vi "Read resource name.vi"(8 "error in (no error)":errorcluster, 11 "FPGATarget in":refnum<class "FPGATarget.lvclass">) -> (0 "error out":errorcluster, 2 "RIO Device":T1, 3 "FPGATarget out":refnum<class "FPGATarget.lvclass">)   [LabVIEW 2013, in "FPGATarget.lvclass"]
uses:
  FPGATarget.lvclass
  <vilib>/userdefined/High Color/nirio_resource_hc.ctl
  FPGATarget.lvclass/FPGATarget.ctl
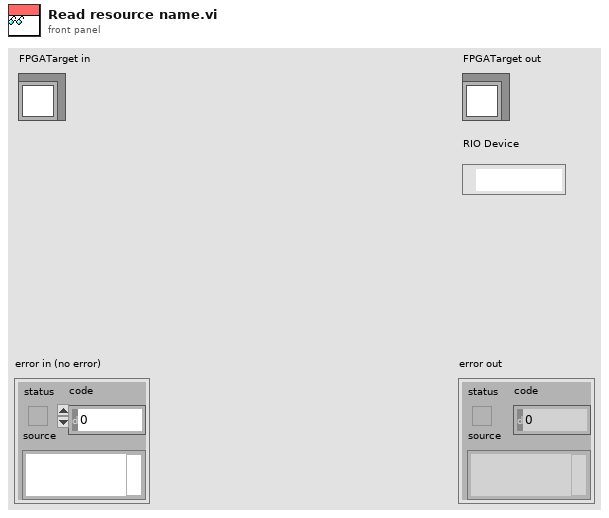
[diagram p1: front panel]
types:
  T1 = typedef "nirio_resource_hc.ctl" = tag
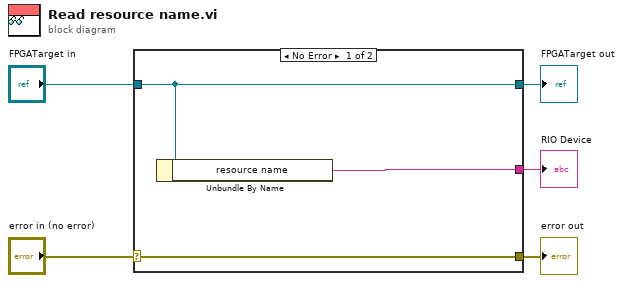
[diagram p0: block diagram]
diagram:
  n1 = case shown="No Error" "error in (no error)" {
    selector: "error in (no error)" -> [w8 w9]
    tunnel: [w8 w9] -> w4
    tunnel: [w7 w10] -> w2
    tunnel: "FPGATarget in" -> [w7 w10]
    tunnel: [w6 _] -> w1
    frame No Error {
      n2 = Unbundle By Name(w7) -> ("resource name"=w6:T1)
    }
    frame Error {
    }
  }
  "error out" <- w4
  "FPGATarget out" <- w2
  "RIO Device" <- w1
